vi "_CSMObj-Remove Chain Node.vi"(8 "Error in":errorcluster caption="Error in (no error)", 10 "Requested Name":string, 11 "CSMObj in":T1={"Requested Name"="", "Module Name"="", "Mode"=enum."Stand Alone", "Queue"=refnum, "CSM-Data"=refnum, "User Event"=refnum, "Status Change Event"=refnum, "Allowed Messages"=[], "Mode-Data"=refnum, "Group Name"="", "Exit Event"=refnum}) -> (0 "Error out":errorcluster, 3 "CSMObj out":T1={"Requested Name"="", "Module Name"="", "Mode"=enum."Stand Alone", "Queue"=refnum, "CSM-Data"=refnum, "User Event"=refnum, "Status Change Event"=refnum, "Allowed Messages"=[], "Mode-Data"=refnum, "Group Name"="", "Exit Event"=refnum})   [LabVIEW 2020, in "Communicable State Machine.lvlib"]
uses:
  Communicable State Machine.lvlib
  _CSMObj.ctl
  Priority Queue.lvclass
  _CSM_MODE.ctl
  _CSMObj-Data.ctl
  _CSM Status Change Event Data.ctl
  _CSMObj-ModeData.ctl
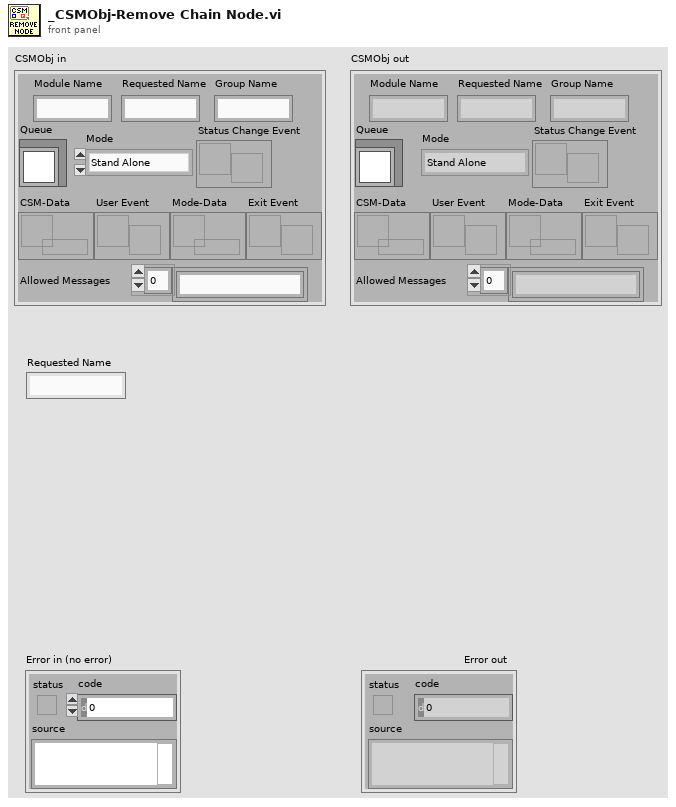
[diagram p1: front panel]
types:
  T1 = typedef "Communicable State Machine.lvlib/_CSMObj.ctl" = cluster{"Requested Name":string, "Module Name":string, "Mode":T2, "Queue":refnum<class "Priority Queue.lvclass">, "CSM-Data":refnum<data-value>, "User Event":refnum<user-event>, "Status Change Event":refnum<user-event>, "Allowed Messages":string[], "Mode-Data":refnum<data-value>, "Group Name":string, "Exit Event":refnum<user-event>}
  T2 = typedef "Communicable State Machine.lvlib/_CSM_MODE.ctl" = enum16{"Not Exist", "Stand Alone", "CSM", "Worker Agent", "Worker", "Chain", "Chain Node"}
  T3 = typedef "Communicable State Machine.lvlib/_CSMObj-ModeData.ctl" = cluster{"Share Count":i32, "Messages of Chain Nodes":cluster{"Module Name":string, "Allowed Messages":string[]}[], "Chain Message Mapping Map":variant}
  T4 = cluster{"Module Name":string, "Allowed Messages":string[]}[]
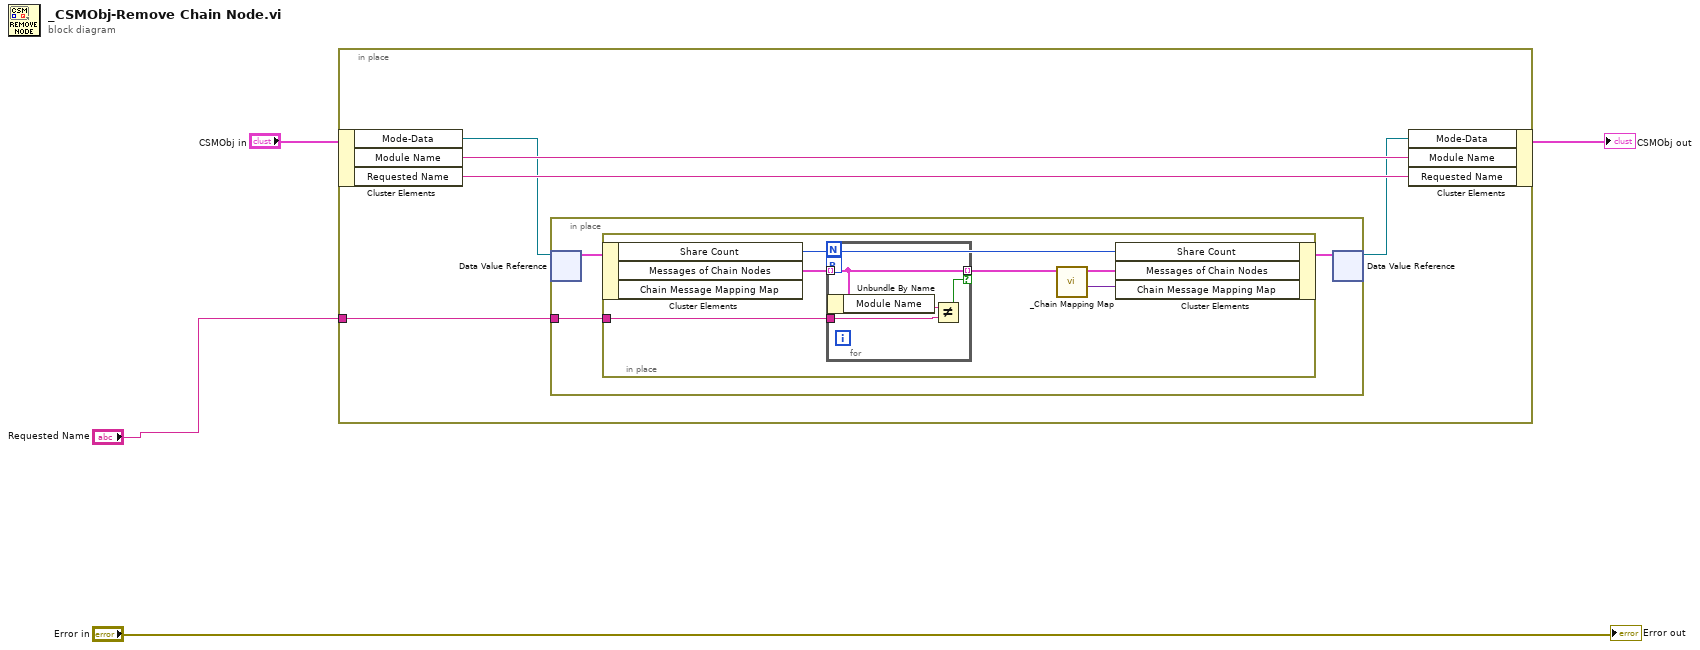
[diagram p0: block diagram]
diagram:
  n1 = in-place "In Place Element Structure" {
    in-place-border: "Requested Name" -> [w5]
    n2 = in-place-cluster #1("CSMObj in") -> ("Mode-Data"=w7:refnum<data-value>, "Module Name"=w9:string, "Requested Name"=w8:string)
    n3 = in-place {
      in-place-border: w5 -> [w10]
      n4 = in-place-dvr #2(w7) -> (w12:T3)  [unwired: 1 out]
      n5 = in-place {
        in-place-border: w10 -> [w14]
        n6 = in-place-cluster #3(w12) -> ("Share Count"=w16:i32, "Messages of Chain Nodes"=w15:T4)  [unwired: 1 out]
        n7 = for {
          tunnel: w15 -> [w22] mode=indexing
          tunnel: [w22] -> w13 mode=indexing if=w19
          tunnel: w14 -> [w20]
          workers-P: _ -> [_]
          n8 = Unbundle By Name(w22) -> ("Module Name"=w21:string)
          n9 = Not Equal?(x=w21, y=w20) -> (x != y?=w19:bool)
        }
        n10 = call "_Chain Mapping Map.vi"("Messages of Chain Nodes"=w13) -> ("variant"=w17:variant, "Messages of Chain Nodes (dup)"=w18:T4)  [unwired: 9 in]
        n11 = in-place-cluster #3("Share Count"=w16, "Messages of Chain Nodes"=w18, "Chain Message Mapping Map"=w17) -> (w11:T3)
      }
      n12 = in-place-dvr #2(w11) -> (w6:refnum<data-value>)  [unwired: 1 out]
    }
    n13 = in-place-cluster #1("Mode-Data"=w6, "Module Name"=w9, "Requested Name"=w8) -> (→"CSMObj out":T1)
  }
  "Error out" <- "Error in"
